vi "4461 - Create IO Channels Parallel Uneven array.vi"(0 "sample mode":i32(ring)=10178 items=["Finite Samples"=10178, "Continuous Samples"=10123], 1 "Channels: Lockin":T1={"REF f (Hz)"=[0.4, 0.4], "REF phi (deg)"=[0.0, 0.0]} {"REF phi (deg)" format="%#_3g"}, 6 "error in":errorcluster, 7 "AI Buffer Size (S)":i32=10, 8 "sampling info":cluster{"Fs":dbl, "#s":dbl}, 9 "AO":T2={"AO amp (V)"=[0.1, 0.09, 0.08, 0.07, 0.06, 0.05, 0.04, 0.03], "AO DC (V)"=[0.0, 0.0, 0.0, 0.0, 0.0, 0.0, 0.0, 0.0], "AO f (Hz)"=[13.0, 13.0, 13.0, 13.0, 13.0, 13.0, 13.0, 13.0], "AO phi (deg)"=[0.0, 0.0, 0.0, 0.0, 0.0, 0.0, 0.0, 0.0], "function"=[enum."Sine Wave", enum."Sine Wave", enum."Sine Wave", enum."Sine Wave", enum."Sine Wave", enum."Sine Wave", enum."Sine Wave", enum."Sine Wave"]} {"AO DC (V)" format="%#_6p"; "AO amp (V)" format="%#_6p"}, 10 "AO Configuration":T3(array[cluster]), 11 "AI Configuration":T4(array[cluster])) -> (2 "AO Task":refnum<k21>[](array[refnum]), 3 "AI task":refnum<k21>[](array[refnum]), 4 "error out":errorcluster, 5 "phase log":dbl[](array[numeric])=[0.99999999999938, 0.99999999999938])   [LabVIEW 2016]
uses:
  <vilib>/DAQmx/configure/timing.llb/DAQmx Timing (Sample Clock).vi
  <resource>/objmgr/daqmx.rc
  <vilib>/DAQmx/read.llb/DAQmx Read (Analog 1D Wfm NChan NSamp).vi
  <vilib>/DAQmx/create/channels.llb/DAQmx Create Channel (AO-Voltage-Basic).vi
  <vilib>/DAQmx/configure/trigger.llb/DAQmx Start Trigger (Digital Edge).vi
  <vilib>/DAQmx/write.llb/DAQmx Write (Analog 1D Wfm NChan NSamp).vi
  <vilib>/DAQmx/create/channels.llb/DAQmx Create Channel (AI-Voltage-Basic).vi
panel:
  out "RefClk.Src":tag
  out "#samp":dbl
  in  "AI.FilterDelay":dbl
  in  "AI.Gain":dbl
  in  "input terminal configuration":i32(ring)=-1 items=["default"=-1, "RSE"=10083, "NRSE"=10078, "Differential"=10106, "Pseudodifferential"=12529]
  in  "output terminal configuration":i32(ring)=-1 items=["Default"=-1, "RSE"=10083, "Differential"=10106, "Pseudodifferential"=12529]
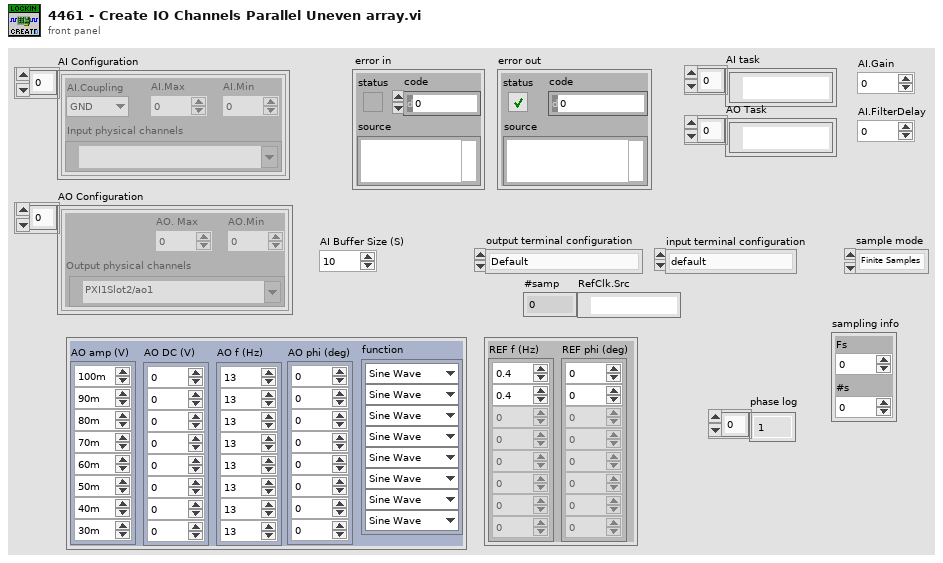
[diagram p1: front panel]
types:
  T1 = cluster{"REF f (Hz)":dbl[], "REF phi (deg)":dbl[]}
  T2 = cluster{"AO amp (V)":dbl[], "AO DC (V)":dbl[], "AO f (Hz)":dbl[], "AO phi (deg)":dbl[], "function":enum16{"Sine Wave", "Triangle Wave", "Square Wave", "Sawtooth Wave"}[]}
  T3 = cluster{"Output physical channels":tag, "AO. Max":dbl, "AO.Min":dbl}[]
  T4 = cluster{"AI.Coupling":enum16{"AC", "DC", "GND"}, "AI.Max":dbl, "AI.Min":dbl, "Input physical channels":tag}[]
  T5 = cluster{"AI.Coupling":enum16{"AC", "DC", "GND"}, "AI.Max":dbl, "AI.Min":dbl, "Input physical channels":tag}
  T6 = cluster{"Output physical channels":tag, "AO. Max":dbl, "AO.Min":dbl}
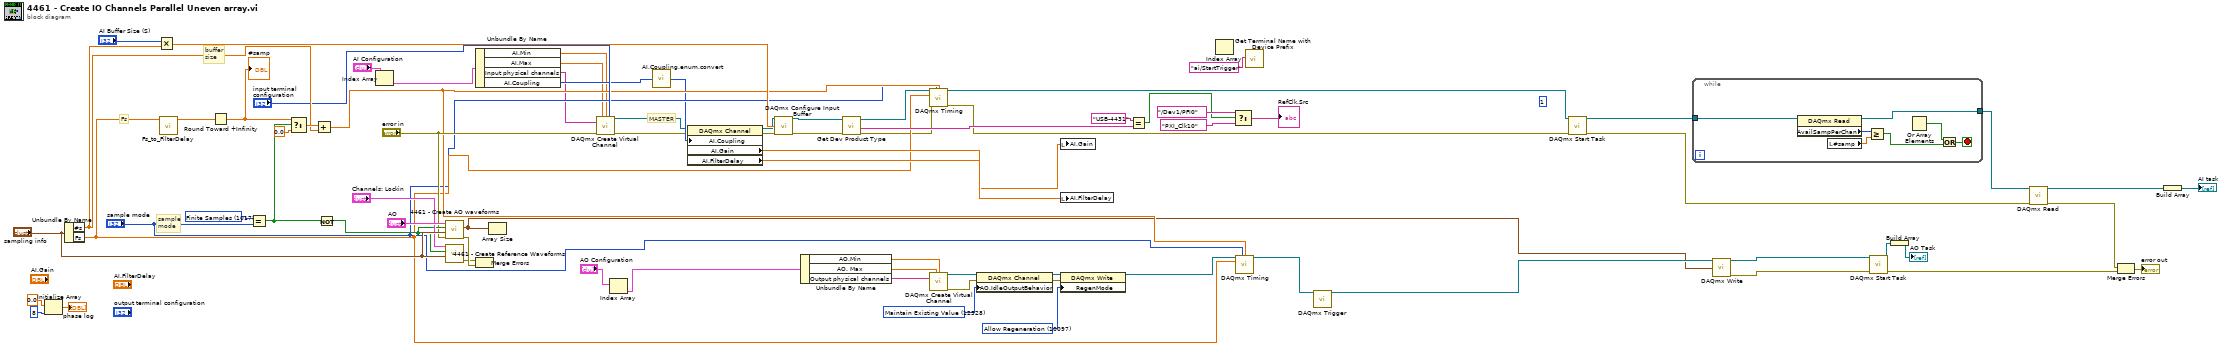
[diagram p0: block diagram]
diagram:
  w8 = 10097 items=["Allow Regeneration"=10097, "Do Not Allow Regeneration"=10158] ("RegenMode")
  w7 = 12528 items=["Zero Volts"=12526, "High-Impedance"=12527, "Maintain Existing Value"=12528] ("AO.IdleOutputBehavior")
  (unwired) 1
  w69 = 10178 items=["Finite Samples"=10178, "Continuous Samples"=10123] ("sample mode 2")
  # "MASTER"
  # "Fs"
  # "sample\nmode"
  # "buffer\nsize"
  n1 = Initialize Array(0.0 ("element"), 8 ("dimension size")) -> (→"phase log":dbl[])
  n2 = Unbundle By Name("sampling info") -> ("#s"=w66:dbl, "Fs"=w46:dbl)
  n3 = Multiply(x="AI Buffer Size (S)", y=w66) -> (x*y=w53:dbl)
  n4 = call "Fs_to_FilterDelay.vi"("Fs"=w46) -> ("Total Filter Delay (samples)"=w72:dbl)  [unwired: 10 in]
  n5 = Round Toward +Infinity(x=w72) -> (ceil(x): smallest int >= x=w62:dbl)
  "#samp" <- w62
  n6 = Equal?(x=w69, y="sample mode") -> (x = y?=w64:bool)
  n7 = Select(t=w62, s=w64, f=0.0) -> (s? t:f=w70:dbl)
  n8 = Add(x=w70, y=w66) -> (x+y=w47:dbl)
  n9 = Not(x=w64) -> (.not. x?=w63:bool)
  n10 = Index Array(array="AI Configuration") -> (element=w19:T5)  [unwired: 1 in]
  n11 = call "4461 - Create AO waveforms.vi"("error in (no error)"="error in", "sampling info"="sampling info", "reset signal"=w63, "AO"="AO") -> ("error out"=w58:errorcluster, "AO Array"=w4:waveform(dbl)[])  [unwired: 4 in, 2 out]
  n12 = call "4461 - Create Reference Waveforms.vi"("sampling info"="sampling info", "reset signal"=w63, "Lockin"="Channels: Lockin") -> ("error out"=w42:errorcluster)  [unwired: 5 in, 3 out]
  n13 = Unbundle By Name(w19) -> ("AI.Min"=w31:dbl, "AI.Max"=w30:dbl, "Input physical channels"=w27:tag, "AI.Coupling"=w32:enum16{"AC", "DC", "GND"})
  n14 = Merge Errors(w42, w58) -> ()  [unwired: 1 out]
  n15 = Array Size(array=w4) -> ()  [unwired: 1 out]
  n16 = call-poly <vilib>:"DAQmx Create Virtual Channel.vi"("maximum value"=w30, "minimum value"=w31, "input terminal configuration"="input terminal configuration", "physical channels"=w27, "error in"="error in") -> ("task out"=w28:refnum<k21>, "error out"=w29:errorcluster)  [unwired: 9 in]
  n17 = Index Array(array="AO Configuration") -> (element=w16:T6)  [unwired: 1 in]
  n18 = call "AI.Coupling.enum.convert.vi"("AI.Coupling"=w32) -> ("Numeric"=w33:i32)
  n19 = property class="DAQmx Channel"(reference=w28, error in=w29, "AI.Coupling"=w33) -> (reference out=w26:refnum<k21>, error out=w23:errorcluster, "AI.Gain"=w55:dbl, "AI.FilterDelay"=w56:dbl)
  n20 = call <vilib>:"DAQmx Configure Input Buffer.vi"("task/channels in"=w26, "buffer size (in samples per channel)"=w53, "error in"=w23) -> ("task out"=w25:refnum<k21>, "error out"=w24:errorcluster)  [unwired: 11 in]
  n21 = Unbundle By Name(w16) -> ("AO.Min"=w13:dbl, "AO. Max"=w14:dbl, "Output physical channels"=w15:tag)
  n22 = call "Get Dev Product Type.vi"("error in (no error)"=w24, "Refnum in"=w25) -> ("error out"=w21:errorcluster, "ProductType"=w52:string, "Refnum out"=w22:refnum<k21>)  [unwired: 7 in]
  n23 = call-poly <vilib>:"DAQmx Timing.vi"("task/channels in"=w22, "sample mode"="sample mode", "samples per channel"=w47, "rate"=w46, "error in"=w21) -> ("task out"=w3:refnum<k21>, "error out"=w37:errorcluster)  [unwired: 9 in]
  n24 = call-poly <vilib>:"DAQmx Create Virtual Channel.vi"("maximum value"=w14, "minimum value"=w13, "physical channels"=w15) -> ("task out"=w12:refnum<k21>, "error out"=w11:errorcluster)  [unwired: 11 in]
  n25 = property class="DAQmx Channel"(reference=w12, error in=w11, "AO.IdleOutputBehavior"=w7) -> (reference out=w10:refnum<k21>, error out=w9:errorcluster)
  n26 = local write "AI.Gain"(w55) -> ()
  n27 = local write "AI.FilterDelay"(w56) -> ()
  n28 = property class="DAQmx Write"(reference=w10, error in=w9, "RegenMode"=w8) -> (reference out=w48:refnum<k21>)  [unwired: 1 out]
  n29 = Equal?(x="USB-4431" ("ProductType"), y=w52) -> (x = y?=w36:bool)
  n30 = Index Array() -> ()  [unwired: 2 in, 1 out]
  n31 = Select(t=tag "/Dev1/PFI0" ("RefClk.Src"), s=w36, f=tag "PXI_Clk10" ("RefClk.Src")) -> (s? t:f=→"RefClk.Src":tag)
  n32 = call-poly <vilib>:"DAQmx Timing.vi"("task/channels in"=w48, "sample mode"="sample mode", "samples per channel"=w47, "rate"=w46) -> ("task out"=w6:refnum<k21>)  [unwired: 10 in, 1 out]
  n33 = call "Get Terminal Name with Device Prefix.vi"("Local Terminal Name"="ai/StartTrigger") -> ()  [unwired: 8 in, 3 out]
  n34 = call-poly <vilib>:"DAQmx Trigger.vi"("task/channels in"=w6) -> ("task out"=w5:refnum<k21>)  [unwired: 13 in, 1 out]
  n35 = call <vilib>:"DAQmx Start Task.vi"("task/channels in"=w3, "error in"=w37) -> ("task out"=w35:refnum<k21>, "error out"=w38:errorcluster)  [unwired: 12 in]
  n36 = while {
    tunnel: w35 -> [w83]
    tunnel: [w80] -> w50
    stop <- w81 stop-if-true
    n37 = property class="DAQmx Read"(reference=w83) -> (reference out=w80:refnum<k21>, "AvailSampPerChan"=w79:u32)  [unwired: 1 in, 1 out]
    n38 = local read "#samp"() -> (w78:dbl)
    n39 = Greater Or Equal?(x=w79, y=w78) -> (x >= y?=w77:bool)
    n40 = Or Array Elements() -> (logical OR=w82:bool)  [unwired: 1 in]
    n41 = Or(x=w82, y=w77) -> (x .or. y?=w81:bool)
  }
  n42 = call-poly <vilib>:"DAQmx Write.vi"("task/channels in"=w5, "data"=w4) -> ("task out"=w44:refnum<k21>, "error out"=w43:errorcluster)  [unwired: 11 in, 1 out]
  n43 = call <vilib>:"DAQmx Start Task.vi"("task/channels in"=w44, "error in"=w43) -> ("task out"=w2:refnum<k21>, "error out"=w40:errorcluster)  [unwired: 12 in]
  n44 = Build Array(w2) -> (→"AO Task":refnum<k21>[])
  n45 = call-poly <vilib>:"DAQmx Read.vi"("task/channels in"=w50, "error in"=w38) -> ("task out"=w49:refnum<k21>, "error out"=w39:errorcluster)  [unwired: 11 in, 1 out]
  n46 = Merge Errors(w39, w40) -> (→"error out":errorcluster)
  n47 = Build Array(w49) -> (→"AI task":refnum<k21>[])
